vi "Custom GZipStream.vi"(1 "Compression Mode":i32(ring)=1 items=["Decompress", "Compress"], 2 "System.IO.Stream":refnum<k24>, 3 "error in (no error)":errorcluster) -> (6 "System.IO.Compression.GZipStream":refnum<k24>, 7 "error out":errorcluster)   [LabVIEW 2018, in "Kompress.lvlib"]
uses:
  Kompress.lvlib
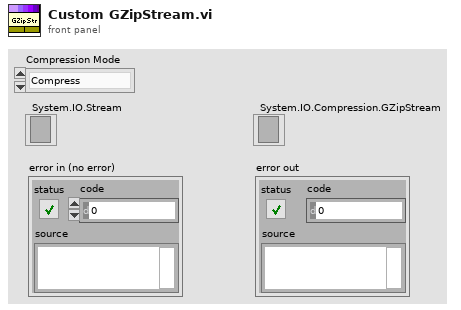
[diagram p1: front panel]
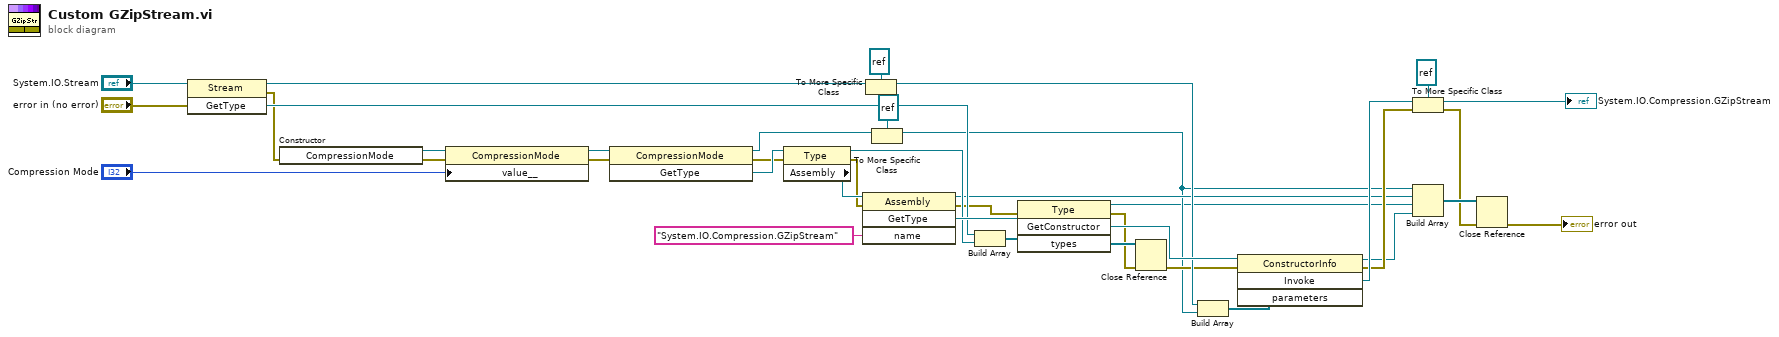
[diagram p0: block diagram]
diagram:
  n1 = invoke class="Stream" method="GetType"(reference="System.IO.Stream", error in="error in (no error)") -> (reference out=w25:refnum<k24>, error out=w2:errorcluster, "GetType"=w30:refnum<k24>)  [unwired: 1 in]
  n2 = constructor class="CompressionMode" ("gs")(error in=w2) -> (reference out=w38:refnum<k24>, error out=w15:errorcluster)  [unwired: 2 in, 1 out]
  n3 = property class="CompressionMode"(reference=w38, error in=w15, "value__"="Compression Mode") -> (reference out=w36:refnum<k24>, error out=w16:errorcluster)
  n4 = invoke class="CompressionMode" method="GetType"(reference=w36, error in=w16) -> (reference out=w26:refnum<k24>, error out=w17:errorcluster, "GetType"=w35:refnum<k24>)  [unwired: 1 in]
  n5 = property class="Type"(reference=w35, error in=w17) -> (reference out=w29:refnum<k24>, error out=w18:errorcluster, "Assembly"=w34:refnum<k24>)
  n6 = invoke class="Assembly" method="GetType"(reference=w34, error in=w18, "name"="System.IO.Compression.GZipStream") -> (reference out=w9:refnum<k24>, error out=w19:errorcluster, "GetType"=w33:refnum<k24>)  [unwired: 1 in, 1 out]
  n7 = To More Specific Class(target class=refnum<k24> refnum ("reference out"), reference=w25) -> (specific class reference=w22:refnum<k24>)  [unwired: 1 in, 1 out]
  n8 = To More Specific Class(target class=refnum<k24> refnum ("reference out"), reference=w26) -> (specific class reference=w8:refnum<k24>)  [unwired: 1 in, 1 out]
  n9 = Build Array(w30, w29) -> (w31:refnum<k24>[])
  n10 = invoke class="Type" method="GetConstructor"(reference=w33, error in=w19, "types"=w31) -> (reference out=w7:refnum<k24>, error out=w20:errorcluster, "GetConstructor"=w28:refnum<k24>, "types"=w27:refnum<k24>[])  [unwired: 1 in]
  n11 = Close Reference(reference=w27, error in (no error)=w20) -> (error out=w14:errorcluster)
  n12 = Build Array(w22, w8) -> (w21:refnum<k24>[])
  n13 = invoke class="ConstructorInfo" method="Invoke"(reference=w28, error in=w14, "parameters"=w21) -> (reference out=w6:refnum<k24>, error out=w10:errorcluster, "Invoke"=w13:refnum<k24>)  [unwired: 1 in, 1 out]
  n14 = To More Specific Class(target class=refnum<k24> refnum ("new reference"), reference=w13, error in=w10) -> (specific class reference=→"System.IO.Compression.GZipStream":refnum<k24>, error out=w4:errorcluster)
  n15 = Build Array(w8, w9, w7, w6) -> (w5:refnum<k24>[])
  n16 = Close Reference(reference=w5, error in (no error)=w4) -> (error out=→"error out":errorcluster)
